vi "Calculate Next Rx Indexes.vi"(9 "message handles":T1 {"Rx status handles" format="%.0x"; "Tx status handles" format="%.0x"; "timestamps" format="%.0x"; "parameters"."RxBC channel handle" format="%.0x"; "parameters"."RxRT channel handle" format="%.0x"; "parameters"."Tx channel handle" format="%.0x"}, 10 "message":T5={"name"="", "message type"="BC to RT", "endpoint Tx"={"terminal address"=0, "subaddress"=0}, "endpoint Rx"={"terminal address"=0, "subaddress"=0}, "create timestamp channel"=FALSE, "mode code"=0, "number of words"=0, "parameters"=[]}, 11 "index":i32) -> (2 "message map value":T4={"value indexes"=[], "message"={"name"="", "message type"="BC to RT", "endpoint Tx"={"terminal address"=0, "subaddress"=0}, "endpoint Rx"={"terminal address"=0, "subaddress"=0}, "create timestamp channel"=FALSE, "mode code"=0, "number of words"=0, "parameters"=[]}, "Tx status count"=0, "Rx status count"=0}, 3 "next index":i32)   [LabVIEW 2020, in "AIM MIL-STD-1553 Engine.lvlib" / "Implementation.lvlib" / "Rx Execution Unit.lvclass"]
uses:
  Rx Execution Unit.lvclass
  Shared/Parameter Definition.ctl
  Shared/Address.ctl
  Shared/Terminal Endpoint.ctl
  Shared/Message Type.ctl
  Shared/Message Definition.ctl
  Message Map Value.ctl
  <vilib>/NI VeriStand/Custom Device API/Custom Device Item Ref.ctl
  <vilib>/NI VeriStand/Custom Device API/Custom Device API.lvlib
  Execution Unit/Parameter Handles.ctl
  Execution Unit/Execution Unit.lvclass
  Execution Unit/Message Handles.ctl
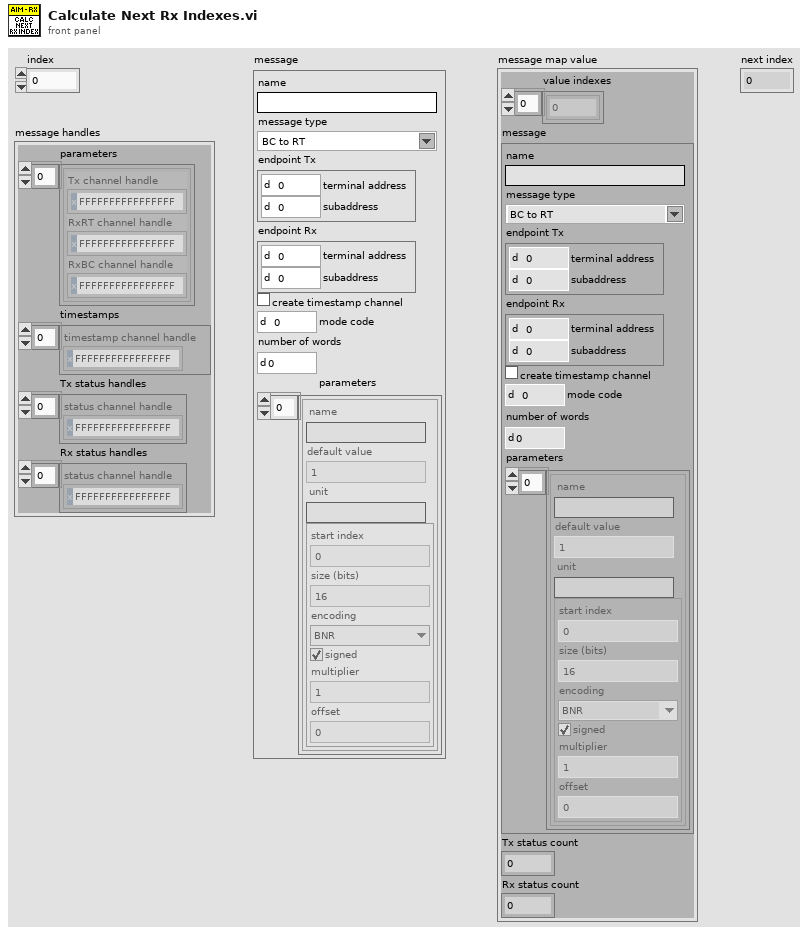
[diagram p1: front panel]
types:
  T1 = typedef "AIM MIL-STD-1553 Engine.lvlib/Implementation.lvlib/Execution Unit.lvclass/Message Handles.ctl" = cluster{"parameters":T2[], "timestamps":T3[], "Tx status handles":T3[], "Rx status handles":T3[]}
  T2 = typedef "AIM MIL-STD-1553 Engine.lvlib/Implementation.lvlib/Execution Unit.lvclass/Parameter Handles.ctl" = cluster{"Tx channel handle":T3, "RxRT channel handle":T3, "RxBC channel handle":T3}
  T3 = typedef "Custom Device API.lvlib/Custom Device Item Ref.ctl" = u64
  T4 = typedef "AIM MIL-STD-1553 Engine.lvlib/Implementation.lvlib/Rx Execution Unit.lvclass/Message Map Value.ctl" = cluster{"value indexes":i32[], "message":T5, "Tx status count":i32, "Rx status count":i32}
  T5 = typedef "Message Definition.ctl" = cluster{"name":string, "message type":T6, "endpoint Tx":T7, "endpoint Rx":T7, "create timestamp channel":bool, "mode code":u16, "number of words":u16, "parameters":cluster{"name":string, "default value":dbl, "unit":string, "parameter definition":T9}[]}
  T6 = typedef "Message Type.ctl" = string
  T7 = typedef "Terminal Endpoint.ctl" = cluster{"terminal address":T8, "subaddress":T8}
  T8 = typedef "Address.ctl" = u16
  T9 = typedef "Parameter Definition.ctl" = cluster{"start index":i32, "size (bits)":i32, "encoding":enum16{"BNR", "BCD", "Discrete"}, "signed":bool, "multiplier":dbl, "offset":dbl}
  T10 = cluster{"name":string, "default value":dbl, "unit":string, "parameter definition":T9}[]
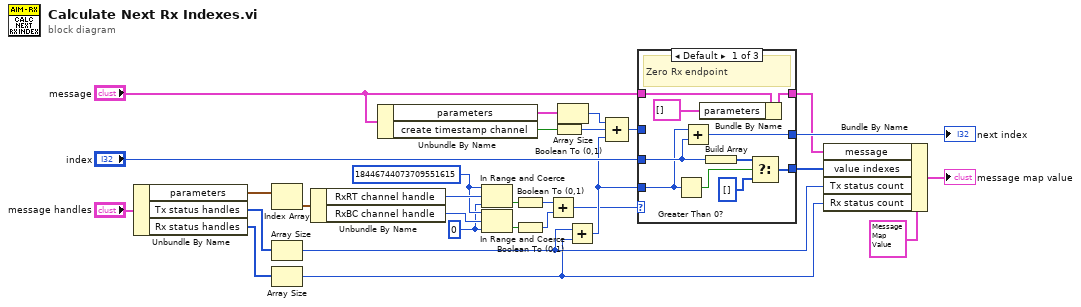
[diagram p0: block diagram]
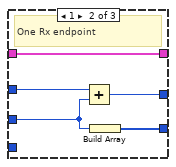
[diagram p2: hidden frame]
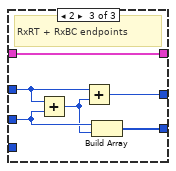
[diagram p3: hidden frame]
diagram:
  w11 = T3 0 ("upper limit")
  w12 = T3 18446744073709551615 ("upper limit")
  n1 = Unbundle By Name("message handles") -> ("parameters"=w5:T2[], "Tx status handles"=w17:T3[], "Rx status handles"=w18:T3[])
  n2 = Index Array(array=w5) -> (element=w21:T2)  [unwired: 1 in]
  n3 = Array Size(array=w17) -> (size(s)=w9:i32)
  n4 = Array Size(array=w18) -> (size(s)=w8:i32)
  n5 = Unbundle By Name(w21) -> ("RxRT channel handle"=w16:T3, "RxBC channel handle"=w15:T3)
  n6 = Unbundle By Name("message") -> ("parameters"=w4:T10, "create timestamp channel"=w28:bool)
  n7 = In Range and Coerce(upper limit=w12, x=w16, lower limit=w11) -> (In Range?=w14:bool)  [unwired: 1 out]
  n8 = In Range and Coerce(upper limit=w12, x=w15, lower limit=w11) -> (In Range?=w13:bool)  [unwired: 1 out]
  n9 = Boolean To (0,1)(Boolean=w14) -> (0, 1=w20:i16)
  n10 = Boolean To (0,1)(Boolean=w13) -> (0, 1=w19:i16)
  n11 = Add(x=w20, y=w19) -> (x+y=w6:i16)
  n12 = Boolean To (0,1)(Boolean=w28) -> (0, 1=w7:i16)
  n13 = Array Size(array=w4) -> (size(s)=w3:i32)
  n14 = Add(x=w9, y=w8) -> (x+y=w22:i32)
  n15 = Compound Arithmetic op=ADD(w3, w7, w22) -> (w27:i32)
  n16 = case shown="Default" w6 {
    tunnel: "index" -> [w38 w42 w50]
    tunnel: [w39 w44 w47] -> w26
    tunnel: [w34 w43 w49] -> w23
    tunnel: w27 -> [_ w41 w46]
    tunnel: w22 -> [w37 _ _]
    tunnel: "message" -> [w32 w40 w45]
    tunnel: [w31 w40 w45] -> w1
    frame Default {
      # "Zero Rx endpoint"
      n17 = Greater Than 0?(x=w37) -> (x > 0?=w36:bool)
      n18 = Add(x=w37, y=w38) -> (x+y=w39:i32)
      n19 = Bundle By Name(cluster=w32, "parameters"=T10 []) -> (w31:T5)
      n20 = Build Array(w38) -> (w35:i32[])
      n21 = Select(t=w35, s=w36, f=i32[] []) -> (s? t:f=w34:i32[])
    }
    frame 1 {
      # "One Rx endpoint"
      n22 = Add(x=w41, y=w42) -> (x+y=w44:i32)
      n23 = Build Array(w42) -> (w43:i32[])
    }
    frame 2 {
      # "RxRT + RxBC endpoints"
      n24 = Add(x=w46, y=w50) -> (x+y=w48:i32)
      n25 = Add(x=w46, y=w48) -> (x+y=w47:i32)
      n26 = Build Array(w50, w48) -> (w49:i32[])
    }
  }
  "next index" <- w26
  n27 = Bundle By Name(cluster=T4 {"value indexes"=[], "message"={"name"="", "message type"="BC to RT", "endpoint Tx"={"terminal address"=0, "subaddress"=0}, "endpoint Rx"={"terminal address"=0, "subaddress"=0}, "create timestamp channel"=FALSE, "mode code"=0, "number of words"=0, "parameters"=[]}, "Tx status count"=0, "Rx status count"=0} ("value"), "message"=w1, "value indexes"=w23, "Tx status count"=w9, "Rx status count"=w8) -> (→"message map value":T4)
